vi "Get Name Library File Path.vi"(11 "_Rename in":refnum<class "_Rename.lvclass">) -> (2 "Name Library File Path":path)   [LabVIEW 2020, in "_Rename.lvlib" / "_Rename.lvclass"]
uses:
  _Rename.lvclass
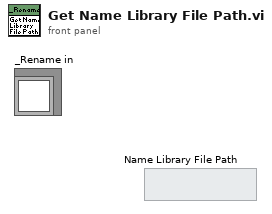
[diagram p1: front panel]
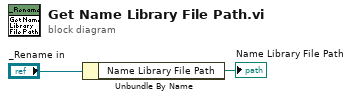
[diagram p0: block diagram]
diagram:
  n1 = Unbundle By Name("_Rename in") -> ("Name Library File Path"=→"Name Library File Path":path)
